vi "Gas_Setup.vi"() -> ()   [LabVIEW 2015]
uses:
  ADAM Controls/Ch_description_ADAM.ctl
  ADAM Controls/Module_type_ADAM.ctl
  ADAM Controls/Function_ADAM.ctl
  ADAM Controls/Channel_State.ctl
  ADAM Controls/Calib_type_ADAM.ctl
  ADAM Controls/Address.ctl
  ADAM Controls/Shut_Off_Valve.ctl
  ADAM Controls/Channel_names.ctl
  Channel_State_Control.ctl
  ADAM Controls/Update_scan_value.ctl
  Anemometry/Anemometry Sub Vis/Globals/Preference_global.vi
panel:
  out "Ch names":string[](array[string])
  in  "Select Plug Ins":bool
  in  "Source Info":string[][](table)
  in  "Carrier 1 Very Low":T1
  in  "Carrier 1 Hi-Tec Range":u16(ring) items=["Very Low", "Low", "High"]
  in  "Trace Hi-Tec Range":u16(ring) items=["5 ml/min", "50 ml/min", "300 ml/min"]
  in  "Carrier 1 High":T1
  in  "Carrier 1 Low":T1
  in  "300 ml/min":T1
  in  "5 ml/min":T1
  in  "Release Orientation":u16(ring) items=["Vertical", "Horizontal 0 Deg", "Downwards", "External System Tests", "Horizontal", "Edit Strings"]
  in  "Source Type":u16(ring) items=["11mm downward facing", "1mm Annulus above tank wall with Internal 2mm Annulus floating roof at 50mm.", "2 x ID=11mm Holes", "23mm IDD=8mm", "2mm Annulus around a quarter of inside of tank wall", "2mm Annulus around inside of tank wall", "4 point source ID=8.5mm located 90 deg apart on 8cm Diameter", "4 x 3mm holes spaced 8mm apart at roof perimeter", "70x70mm", "8  x 3mm holes spaced 10mm apart at roof perimeter", "8mm Annulus around inside of tank wall", "B2 D=6.8mm", "B204 Height 244mm ID 5.5mm", "B230 Height 152.4mm ID 8.5mm", "B30 Area", "B311 ID=11mm", "B331 ID=5.4mm", "B38_8mm_ID_passive", "B38_OD=3.1mm_ID=2mm", "B548 OD=13.8mm ID=3.5mm", "Both_Scrubbers_ID=4mm", "Both_Scrubbers_ID=7mm", "Capped release D=10mm H=10mm Slot=2mm", "D=12mm", "D=13.6mm", "D=16mm (ID=12 mm)", "D=18mm", "D=20mm", "D=22.5mm", "D=3.4mm", "D=5mm (ground release)", "D=6mm (ID=4.2 mm)", "D=7.1mm", "D=9mm", "D=9mm  20mm long passive", "Dext = 8.5 mm", "Exit Port of Solenoid Valve", "H=25:W=100mm", "H=50", "ID=1.6 OD=1.9", "ID=1.9 OD=3.0mm", "ID=103mm", "ID=15 mm 90 deg bend copper tube", "ID=20mm", "ID=24mm", "ID=3.4mm  OD= 4mm", "ID=3.9mm OD=6.3mm", "ID=4.25mm", "ID=4mm", "ID=5.1mm OD=5.8mm (Ground release)", "ID=5.1mm OD=5.8mm (roof release)", "ID=5.1mm at Z= 10mm  (Ground release)", "ID=50mm", "ID=5mm OD=5.8mm", "ID=6mm", "ID=6mm OD=8mm", "ID=7.75mm OD=10mm", "ID=8.6mm", "ID=8mm OD=9mm", "ID=9.2mm", "ID=9.5mm OD=12.5mm", "ID=9mm OD=10mm  Short Passive", "Line Source 100mm  1.07m width", "Line Source 25mm  1.3m long  perp to flow", "Line Source 25x1300", "Line Source 50mm  1.07m Wide", "Line source parallel to flow", "None", "Permeability_rig", "Pond_No1&2_140mm", "Pond_No1&2_84mm", "Pond_No1_84mm", "Pond_No2_84mm", "ROSE 9mm at last grid", "SAV ID=3.5mm", "Sample tubes in source", "Single 5mm Stack", "Single 7.9 mm stack", "THORP  ID=5.1mm", "Twin 5mm Stacks", "Twin Passive Stacks ID=8mm OD=8.7mm", "UKAEA ID=1.7mm", "W=50mm", "Edit Strings"]
  in  "Current Release Temp":dbl format="%.2f"
  in  "Release Temperature":u16(ring) items=["Enter Value", "A_Tunnel:Trav:1", "A_Tunnel:Speed:Dem Velocity", "A_Tunnel:Speed:Calib Tweak", "A_Tunnel:Speed:Dem Voltage", "A_Tunnel:Motor:Temp", "A_Tunnel:Motor:Enable", "A_Tunnel:Turbine:Enable", "A_Tunnel:Turbine_1:Dem_Volts", "A_Tunnel:Turbine_1:Dem_RPM", "Aero_Tunnel:Server:Pulse", "Aero_Tunnel:Motor:Temp", "Aero_Tunnel:Balance:Lift", "Aero_Tunnel:Balance:Pitch", "Aero_Tunnel:Balance:Drag", "Aero_Tunnel:Balance:Side-Force", "Aero_Tunnel:Balance:Yaw", "Aero_Tunnel:Balance:Roll", "B_Tunnel:Motor:Temp", "Cluster Room:General:Temp", "Cluster Room:Temp:Warning", "Complete:Scan:Period", "D_Tunnel:Motor:Temp", "EnFlo Lab:Hygrometry:Rel Humidity", "EnFlo Lab:Hygrometry:Dew Point temp", "EnFlo Lab:Hygrometry:Air Temp", "EnFlo Lab:labstrat1:Z=0m Floor", "EnFlo Lab:labstrat1:Z=0.1m", "EnFlo Lab:labstrat1:Z=0.5m", "EnFlo Lab:labstrat1:Z=1.5m", "EnFlo Lab:labstrat1:Z=2.5m", "EnFlo Lab:labstrat1:Z=3.5m", "EnFlo Lab:labstrat1:Z=4.5m", "EnFlo Lab:labstrat1:Z=5.75m Roof", "EnFlo Lab:labstrat1:Delta T", "EnFlo Lab:Desired:Air Temp", "EnFlo Lab:Heat:Extraction", "EnFlo Lab:labstrat1:Av Temp", "EnFlo Lab:Comp Air:Pressure", "EnFlo Lab:Emergency_Stop:Happy", "EnFlo Lab:Leak_Detector:Happy", "EnFlo Lab:Comp Air:Warning", "EnFlo_Tunnel:Speed:Dem Velocity", "EnFlo_Lab:Ventilation:Enable", "EnFlo_Lab:Window_Fans:Enable", "EnFlo_Lab:Window:Enable", "EnFlo_Lab:Window:Open", "EnFlo_Lab:West Window:Open1", "EnFlo_Lab:West Window:Open2", "EnFlo_Tunnel:Speed:Calib Tweak", "EnFlo_Tunnel:Speed:Dem Current", "EnFlo_Tunnel:Usonic:Velocity", "EnFlo_Tunnel:Usonic Y-ve Duct:Velocity", "EnFlo_Tunnel:Shaft:rpm", "EnFlo_Tunnel:Reference:Velocity", "EnFlo_Tunnel:Ref Pitot Pdyn SDP610:(Pa)", "EnFlo_Tunnel:Ref Pitot Zero SDP610:(Pa)", "EnFlo_Tunnel:Ref Pitot Zero:Enable", "EnFlo_Tunnel:Ref Pitot:Z (mm)", "EnFlo_Tunnel:Ref Pitot:Velocity", "EnFlo_Tunnel:Hydrosonic:Integral", "EnFlo_Tunnel:Days Run at:2.5m/s", "EnFlo_Tunnel:Floor_Cooling:Enable", "EnFlo_Tunnel:Heat_Ex_Div_Valve:Dem Pos", "EnFlo_Tunnel:Exit Duct:Dem Temp", "EnFlo_Tunnel:Exit Duct Top:Temp", "EnFlo_Tunnel:Exit Duct:Temp", "EnFlo_Tunnel:Chilled Water:Motor1 Temp", "EnFlo_Tunnel:Chilled Water:Motor2 Temp", "EnFlo_Tunnel:Chilled Water:Pressure_OK", "EnFlo_Tunnel:Chilled Water:Supply", "EnFlo_Tunnel:Chilled Water:Return", "EnFlo_Tunnel:Chilled Water:Dem Temp", "EnFlo_Tunnel:Chiller_Pump:Enable", "EnFlo_Tunnel:Chiller_Pump:Running", "EnFlo_Tunnel:Chilled Water:Valve Dem Pos", "EnFlo_Tunnel:Chilled Water:Valve Dem Voltage", "EnFlo_Tunnel:Chilled Water:Pressure_return (Bar)", "EnFlo_Tunnel:Chilled Water:Motor_Dem_Voltage", "EnFlo_Tunnel:Chilled Water:Desired_Delta_P", "EnFlo_Tunnel:Chilled Water:Pressure_supply (Bar)", "EnFlo_Tunnel:Fan Gearbox:Y+ Temp", "EnFlo_Tunnel:Fan Gearbox:Y- Temp", "EnFlo_Tunnel:Heater:Enable", "EnFlo_Tunnel:Motor:Enable", "EnFlo_Tunnel:Warning_Cone:Enable", "EnFlo_Tunnel:Tap_Water:Enable", "EnFlo_Tunnel:Pressure:Static", "EnFlo_Tunnel:P1:Enable", "EnFlo_Tunnel:P2:Enable", "EnFlo_Tunnel:P3:Enable", "EnFlo_Tunnel:P4:Enable", "EnFlo_Tunnel:P5:Enable", "EnFlo_Tunnel:K_Factor:1st_Honeycomb", "EnFlo_Tunnel:K_Factor:1st_Screen", "EnFlo_Tunnel:K_Factor:2nd_Screen", "EnFlo_Tunnel:K_Factor:2nd_Honeycomb_Heaters_Screen", "EnFlo_Tunnel:Inlet_Fan:Front_Trunk", "EnFlo_Tunnel:Inlet_Fan:Y-ve", "EnFlo_Tunnel:Inlet_Fan:Y+ve", "EnFlo_Tunnel:Inlet_Fan:Above Y-ve", "EnFlo_Tunnel:Inlet_Fan:Above Y=550", "EnFlo_Tunnel:Inlet_Fan:Above Y=1650", "EnFlo_Tunnel:Inlet_Fan:Upwards", "EnFlo_Tunnel:Motor:Temp", "EnFlo_Tunnel:Trav Origin:X Offset", "EnFlo_Tunnel:Trav Pos:X", "EnFlo_Tunnel:Trav Pos:Y", "EnFlo_Tunnel:Trav Pos:Z", "EnFlo_Tunnel:Temp:Pre_Inlet_Y=1500_Z=450", "EnFlo_Tunnel:Temp:Pre_Inlet_Y=-1500_Z=450", "EnFlo_Tunnel:Temp:Pre_Inlet_Y=1000_Z=450", "EnFlo_Tunnel:Temp:Pre_Inlet_Y=-1000_Z=450", "EnFlo_Tunnel:Temp:Pre_Inlet_Y=500_Z=450", "EnFlo_Tunnel:Temp:Pre_Inlet_Y=-500_Z=450", "EnFlo_Tunnel:Temp:Pre_Inlet_Y=0_Z=50", "EnFlo_Tunnel:Temp:Pre_Inlet_Y=0_Z=450", "EnFlo_Tunnel:Temp:Pre_Inlet_Y=0_Z=950", "EnFlo_Tunnel:Temp:Pre_Inlet_Y=0_Z=1450", "EnFlo_Tunnel:Temp:Pre_Inlet_Average", "EnFlo_Tunnel:Temp:Inlet_Y=0_Z=1450", "EnFlo_Tunnel:Temp:Inlet_Y=0_Z=1350", "EnFlo_Tunnel:Temp:Inlet_Y=0_Z=1250", "EnFlo_Tunnel:Temp:Inlet_Y=0_Z=1150", "EnFlo_Tunnel:Temp:Inlet_Y=0_Z=1050", "EnFlo_Tunnel:Temp:Inlet_Y=0_Z=950", "EnFlo_Tunnel:Temp:Inlet_Y=0_Z=850", "EnFlo_Tunnel:Temp:Inlet_Y=0_Z=750", "EnFlo_Tunnel:Temp:Inlet_Y=0_Z=650", "EnFlo_Tunnel:Temp:Inlet_Y=0_Z=550", "EnFlo_Tunnel:Temp:Inlet_Y=0_Z=450", "EnFlo_Tunnel:Temp:Inlet_Y=0_Z=350", "EnFlo_Tunnel:Temp:Inlet_Y=0_Z=250", "EnFlo_Tunnel:Temp:Inlet_Y=0_Z=150", "EnFlo_Tunnel:Temp:Inlet_Y=0_Z=50", "EnFlo_Tunnel:Temp:Inlet_Y=-1500_Z=1450", "EnFlo_Tunnel:Temp:Inlet_Y=-1500_Z=1350", "EnFlo_Tunnel:Temp:Inlet_Y=-1500_Z=1250", "EnFlo_Tunnel:Temp:Inlet_Y=-1500_Z=1150", "EnFlo_Tunnel:Temp:Inlet_Y=-1500_Z=1050", "EnFlo_Tunnel:Temp:Inlet_Y=-1500_Z=950", "EnFlo_Tunnel:Temp:Inlet_Y=-1500_Z=850", "EnFlo_Tunnel:Temp:Inlet_Y=-1500_Z=750", "EnFlo_Tunnel:Temp:Inlet_Y=-1500_Z=650", "EnFlo_Tunnel:Temp:Inlet_Y=-1500_Z=550", "EnFlo_Tunnel:Temp:Inlet_Y=-1500_Z=450", "EnFlo_Tunnel:Temp:Inlet_Y=-1500_Z=350", "EnFlo_Tunnel:Temp:Inlet_Y=-1500_Z=250", "EnFlo_Tunnel:Temp:Inlet_Y=-1500_Z=150", "EnFlo_Tunnel:Temp:Inlet_Y=-1500_Z=50", "EnFlo_Tunnel:Temp:Inlet_Y=-1000_Z=50", "EnFlo_Tunnel:Temp:Inlet_Y=-500_Z=50", "EnFlo_Tunnel:Temp:Inlet_Y=500_Z=50", "EnFlo_Tunnel:Temp:Inlet_Y=1000_Z=50", "EnFlo_Tunnel:Temp:Inlet_Y=1500_Z=50", "EnFlo_Tunnel:Temp:Inlet_Y=-1000_Z=450", "EnFlo_Tunnel:Temp:Inlet_Y=-500_Z=450", "EnFlo_Tunnel:Temp:Inlet_Y=500_Z=450", "EnFlo_Tunnel:Temp:Inlet_Y=1000_Z=450", "EnFlo_Tunnel:Temp:Inlet_Y=1500_Z=450", "EnFlo_Tunnel:Temp:Inlet_Y=-1000_Z=950", "EnFlo_Tunnel:Temp:Inlet_Y=-500_Z=950", "EnFlo_Tunnel:Temp:Inlet_Y=500_Z=950", "EnFlo_Tunnel:Temp:Inlet_Y=1000_Z=950", "EnFlo_Tunnel:Temp:Inlet_Y=1500_Z=950", "EnFlo_Tunnel:Temp:Inlet_Y=-1000_Z=1450", "EnFlo_Tunnel:Temp:Inlet_Y=-500_Z=1450", "EnFlo_Tunnel:Temp:Inlet_Y=500_Z=1450", "EnFlo_Tunnel:Temp:Inlet_Y=1000_Z=1450", "EnFlo_Tunnel:Temp:Inlet_Y=1500_Z=1450", "EnFlo_Tunnel:Inlet_Temp:Average", "EnFlo_Tunnel:Inlet_Temp:St Deviation", "EnFlo_Tunnel:Temp:Floor_Near_1", "EnFlo_Tunnel:Temp:Floor_Near_2", "EnFlo_Tunnel:Temp:Floor_Far_2", "EnFlo_Tunnel:Temp:Floor_Near_3", "EnFlo_Tunnel:Temp:Floor_Far_3", "EnFlo_Tunnel:Temp:Floor_Near_4", "EnFlo_Tunnel:Temp:Floor_Far_4", "EnFlo_Tunnel:Temp:Floor_Near_5", "EnFlo_Tunnel:Temp:Floor_Far_5", "EnFlo_Tunnel:Temp:Floor_Near_6", "EnFlo_Tunnel:Temp:Floor_Far_6", "EnFlo_Tunnel:Temp:Floor_Near_7", "EnFlo_Tunnel:Temp:Floor_Far_7", "EnFlo_Tunnel:Temp:Floor_Near_8", "EnFlo_Tunnel:Temp:Floor_Far_8", "EnFlo_Tunnel:Temp:Floor_Near_12", "EnFlo_Tunnel:Temp:Floor_Far_12", "EnFlo_Tunnel:Temp:Z=50_Y=1415", "EnFlo_Tunnel:Therm:Master_Reference", "EnFlo_Tunnel:Temp:Floor_11.3", "EnFlo_Tunnel:Temp:Floor_12.1", "EnFlo_Tunnel:Temp:Y+ve_Side_Top", "EnFlo_Tunnel:Temp:Y+ve_Side_Middle", "EnFlo_Tunnel:Temp:Y+ve_Side_Bottom", "EnFlo_Tunnel:Temp:Y-ve_Side_Top", "EnFlo_Tunnel:Temp:Y-ve_Side_Middle", "EnFlo_Tunnel:Temp:Y-ve_Side_Bottom", "EnFlo_Tunnel:Temp:Y+ve_Side_Flow_Top", "EnFlo_Tunnel:Temp:Y+ve_Side_Flow_Middle", "EnFlo_Tunnel:Temp:Y+ve_Side_Flow_Bottom", "EnFlo_Tunnel:Temp:Y-ve_Side_Flow_Top", "EnFlo_Tunnel:Temp:Y-ve_Side_Flow_Middle", "EnFlo_Tunnel:Temp:Y-ve_Side_Flow_Bottom", "EnFlo_Tunnel:Temp:Roof_Far_2", "EnFlo_Tunnel:Temp:Roof_Near_3", "EnFlo_Tunnel:Temp:Roof_Far_4", "EnFlo_Tunnel:Temp:Roof_Far_6", "EnFlo_Tunnel:Temp:Roof_Near_7", "EnFlo_Tunnel:Temp:Roof_Far_8", "EnFlo_Tunnel:Temp:Roof_Far_10", "EnFlo_Tunnel:Temp:Roof_Near_12", "EnFlo_Tunnel:Temp:Roof_Far_15", "EnFlo_Tunnel:Temp:Roof_Far_19", "EnFlo_Tunnel:Temp:LDA Probe", "EnFlo_Tunnel:Cold_Wire:Therm", "EnFlo_Tunnel:FFID:Temp", "EnFlo_Tunnel:FFID2:Temp", "Spirit_Smoke:Generator:Enable", "Spirit_Smoke:Generator Puff:Enable", "EnFlo_Tunnel:Lights:Enable", "EnFlo_Tunnel:Trav1 Pos:Z", "EnFlo_Tunnel:Trav1 Pos:Y", "EnFlo_Tunnel:Trav1 Pos:X", "EnFlo_Tunnel:Trav2 Pos:Z", "EnFlo_Tunnel:Trav2 Pos:Y", "EnFlo_Tunnel:Trav2 Pos:X", "EnFlo_Tunnel:Source_Pos:Z", "EnFlo_Tunnel:Safety_Loop:Status", "EnFlo_Tunnel:Gas Solenoid:Status", "EnFlo_Tunnel:Source1:Enable", "EnFlo_Tunnel:Source2:Enable", "EnFlo_Tunnel:Source3:Enable", "EnFlo_Tunnel:Source_Pos:X_Model", "EnFlo_Tunnel:Source_Pos:Y_Model", "EnFlo_Tunnel:Job:Name", "EnFlo_Tunnel:Obstacle/:Building", "EnFlo_Tunnel:Vorticity:Generators", "EnFlo_Tunnel:Roughness:Height", "EnFlo_Tunnel:Side Wall:Separation", "EnFlo_Tunnel:Safety:GMU_Watchdog", "FFID:System:Enable", "Froude:NPL:Atmos_Press", "GMU:Source:Type", "GMU:Release:Orientation", "GMU:Trace:Gas", "GMU:Carrier 1:Gas", "GMU:Carrier 2:Gas", "GMU:Carrier 1:Hi-Tec Range", "GMU:Trace:Hi-Tec Range", "GMU:Carrier 1:Dem Volt", "GMU:Carrier 2:Dem Volt", "GMU:Trace:Dem Volt", "Clean_Air:Hi-Tec:Dem Volt", "GMU:Carrier 1:Meas Volt", "GMU:Carrier 2:Meas Volt", "GMU:Trace:Meas Volt", "Clean_Air:Hi-Tec:Meas Volt", "GMU:Carrier 1:Meas Q", "GMU:Carrier 2:Meas Q", "GMU:Trace:Meas Q", "GMU:Carrier 1:Meas M_dot", "GMU:Carrier 2:Meas M_dot", "GMU:Trace:Meas M_dot", "GMU:Remaining:Nitrogen", "GMU:Remaining:Helium", "GMU:Remaining:CO2", "GMU:Remaining:Krypton", "GMU:Remaining:Ethane", "GMU:Remaining:Propane", "GMU:Calibration:Gas 1", "GMU:Calibration:Gas 2", "GMU:Carrier 1:Dem Q", "GMU:Carrier 2:Dem Q", "GMU:Trace:Dem Q", "GMU:Source:Dem Q", "GMU:Source:Meas Q", "GMU:Source:Meas M_dot", "GMU:Source:Meas Density", "GMU:Source:Meas Den Ratio", "GMU:Source:Dem Strength", "GMU:Source:ppm/%Density", "GMU:Source:Meas Strength", "GMU:Source:Est Time", "GMU:Detector:Meas Current", "GMU:Detector:Strength", "GMU:Test:Ethane trip", "GMU:Source:Release Temp", "GMU:Gas:Enable", "GMU:Detector:Happy", "GMU:Source:Pressure", "GMU:Trace:Open", "GMU:CO2_Rig:Enable", "GMU:CO2_Supply:Pressure (Bar)", "GMU:CO2_Bath:Temp", "GMU:Mixing_Pipe:Temp", "Hydrosonic:Transducer:Setting", "Hydrosonic:Seeder:Enable", "Laser:Power Meter:Reading (mW)", "LDA1:System:Enable", "LDA2:Tank:Supply Temp", "LDA2:System:Enable", "Uni:Chilled Water:Temp", "University:Outside:Temp", "University:Chilled Water:Requested", "A_Tunnel:Probe:Roll", "A_Tunnel:Pitot:Velocity", "A_Tunnel::Velocity", "A_Tunnel:Probe:Yaw", "A_Tunnel:Probe:Pitch", "EnFlo Lab:ScaniValve:Combined_Position", "A_Tunnel:Wing:Pitch", "EnFlo_Tunnel:Seeder_Pump:Enable", "EnFlo_Tunnel:Seeder:High_Flow", "EnFlo_Tunnel:Seeder:Low_Flow", "EnFlo_Tunnel:Seeder_Fridge:Temp", "EnFlo_Tunnel:Seeder:Power", "GMU:Source:Gas", "Tank:Depth:mm", "Tank:Fill_Valve:Enable", "Tank:Fill:Now", "Tank:Desired_Depth:mm", "Tank:Water:Temp", "GMU:CO2_Low:Siren", "A_Tunnel:Trav Pos:Z", "A_Tunnel:Trav Pos:Y", "A_Tunnel:Trav Pos:X", "EnFlo_Stack:Floor:Surface (mm)", "EnFlo Lab:Hygrometry:Rel Humidity_PN", "EnFlo Lab:Hygrometry:Atmos_Press_PN", "EnFlo Lab:Hygrometry:Air Temp_PN", "EnFlo Lab:Hygrometry:Dew Point temp_PN", "EnFlo_Tunnel Metadata:Probe_Setup:Time", "GMU:Source:Live", "GMU:Back_Press_Valve:Volts", "GMU:Back_Press_Valve:Position", "EnFlo_Tunnel:Usonic_Ref_3:Velocity", "EnFlo_Tunnel:Usonic_Ref_3:Direction", "EnFlo_Tunnel:Temp:Pre_Inletx_Ch1", "EnFlo_Tunnel:Trav3 Pos:X", "EnFlo_Tunnel:Trav3 Pos:Z", "EnFlo_Tunnel:Trav3 Pos:Y", "EnFlo_Lab:Window_Fans:Power_%", "EnFlo_Tunnel:Trav_Blockage_Fans:Desired_Volts", "EnFlo_Tunnel:Trav_Blockage_Fans:Meas_Volts", "EnFlo_Tunnel:Trav_Blockage_Fans:Demand_%", "EnFlo_Tunnel:Heater:Dem Volts", "EnFlo_Tunnel:Heater:Dem Power", "EnFlo_Tunnel:Wind:Direction Deg", "EnFlo_Tunnel:Chiller_Pump_Floor:Dem_Power(%)", "EnFlo_Tunnel:Chiller_Pump_Exchanger:Dem_Power(%)", "EnFlo_Tunnel:Exit_Heaters:Dem_Power(%)", "EnFlo_Tunnel Metadata:Screens_Downstream:of Heaters", "EnFlo_Tunnel Metadata:Roughness Elements:1st Row X(m)", "EnFlo_Tunnel:Wind_Turbine:Enable", "EnFlo_Tunnel:De-humidifier:Current_Clamp", "A_Tunnel:Heater_Mat:Enable", "EnFlo_Tunnel:Trav4 Pos:Z", "EnFlo_Tunnel Metadata:2nd_Honeycombe:Upstream of heaters", "GMU:Mains Divertor:Valve", "Status:of:Post_Processing_Machine", "Status:of:ADAM_Server", "Status:of:EnFlo_Tunnel", "Status:of:Aero_Tunnel", "Status:of:A_Tunnel", "EnFlo_Tunnel:Source:Status", "GMU:Trace_2:Dem Volt", "GMU:Trace_2:Meas Volt", "Status:of:Paul_Hayden_Desk"]
  in  "Gas Remaining":string[][](table)
  in  "Calib 2":dbl format="%.2f"
  in  "Calib 1":dbl format="%.2f"
  in  "Carrier 2 Gas":u16(ring) items=["Air", "Nitrogen", "Helium", "CO2", "Krypton", "None"]
  in  "Trace Gas":u16(ring) items=["Propane", "Ethane"]
  in  "Carrier 1 Gas":u16(ring) items=["Air", "Nitrogen", "Helium", "CO2", "Krypton", "None"]
  out "Numerical Values":dbl[](array[numeric]) format="%.9f"
  out "Ch Description Array":T2[](array[typedef]) {"Duty" format="%.0b"; "D" format="%#_5g"; "C" format="%#_5g"; "B" format="%#_5g"; "A" format="%#_5g"}
  out "dup reference":refnum<vi>
  in  "stop":bool
  in  "OK":bool
  # "Calibration Gas (ppm)"
  # "300\nml/min"
  # "5\nml/min"
  # "50\nml/min"
  # "Low\nRange"
  # "Very\nLow\nRange"
  # "High\nRange"
  # "Dispersion Setup"
  # "To Source"
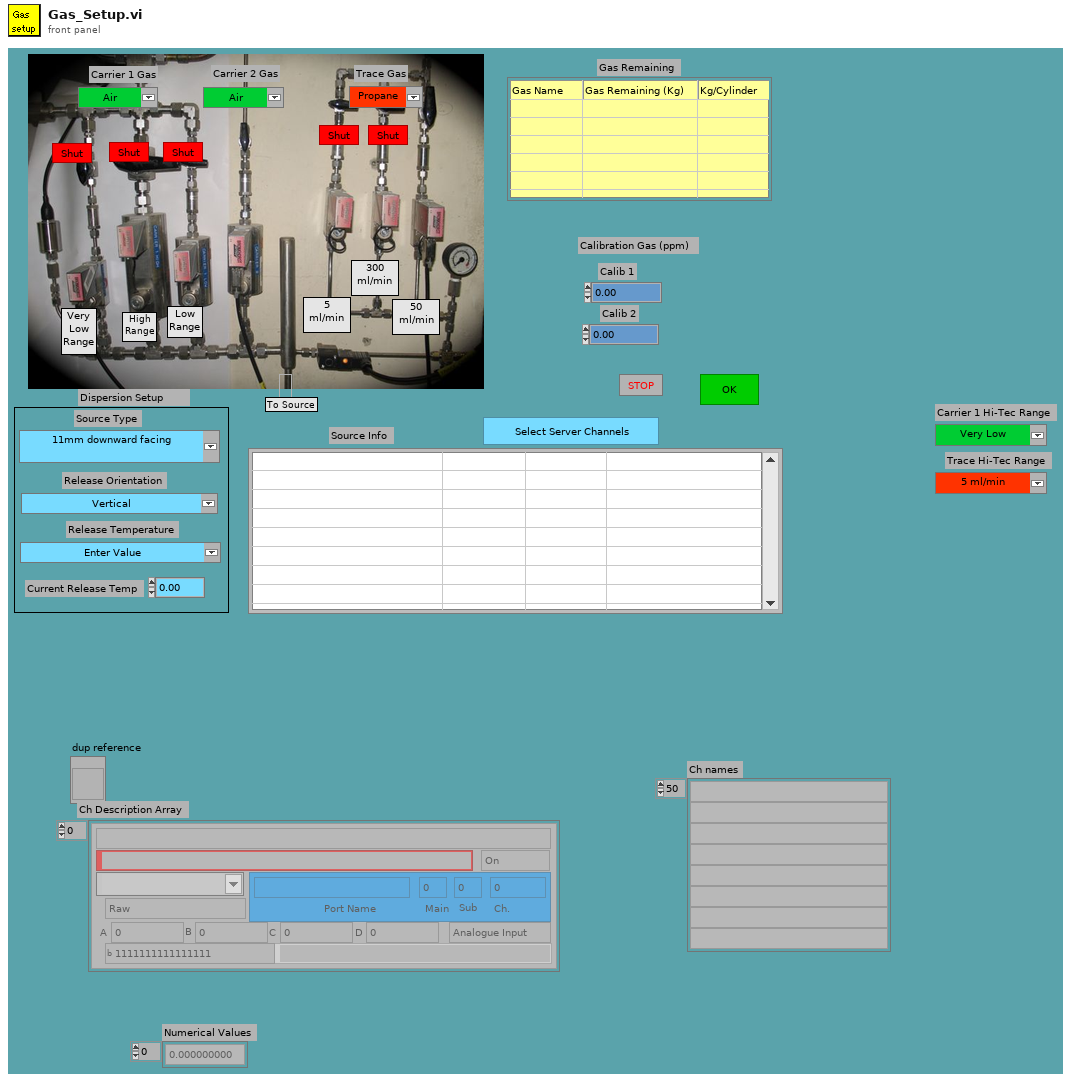
[diagram p1: front panel]
types:
  T1 = typedef "Shut_Off_Valve.ctl" = bool
  T2 = typedef "Ch_description_ADAM.ctl" = cluster{"Ch Name":string, "Type":T3, "Function":T4, "Ch State":T5, "Calibration type":T6, "A":dbl, "B":dbl, "C":dbl, "D":dbl, "Comments":string, "Address":T7, "String":string, "Duty":u16}
  T3 = typedef "Module_type_ADAM.ctl" = string
  T4 = typedef "Function_ADAM.ctl" = enum16{"Analogue Input", "Digital Input", "Event counter", "Event rate", "Analogue Output", "Digital Output", "Relay Output"}
  T5 = typedef "Channel_State.ctl" = enum16{"On", "Off", "Always On", "Always Off"}
  T6 = typedef "Calib_type_ADAM.ctl" = enum16{"Raw", "Bx + A", "Cx^2 + Bx + A", "Dx^3 + Cx^2 + Bx + A", "In Band", "Hi-Tec Q", "Hi-Tec M_dot", "Text"}
  T7 = typedef "Address.ctl" = cluster{"Main":i32, "Ch.":i32, "Sub":i32, "Port Name":string}
  T8 = typedef "Channel_names.ctl" = enum16{"Active Only", "Active + Off", "All Channels"}
  T9 = typedef "Channel_State_Control.ctl" = enum16{"Channel Name", "Channel Name Starts with", "Main Address"}
  T10 = typedef "Update_scan_value.ctl" = cluster{"Channel Name":string, "New Value":dbl}
  T11 = enum16{"Zero or one", "One", "Zero or more", "One or more"}
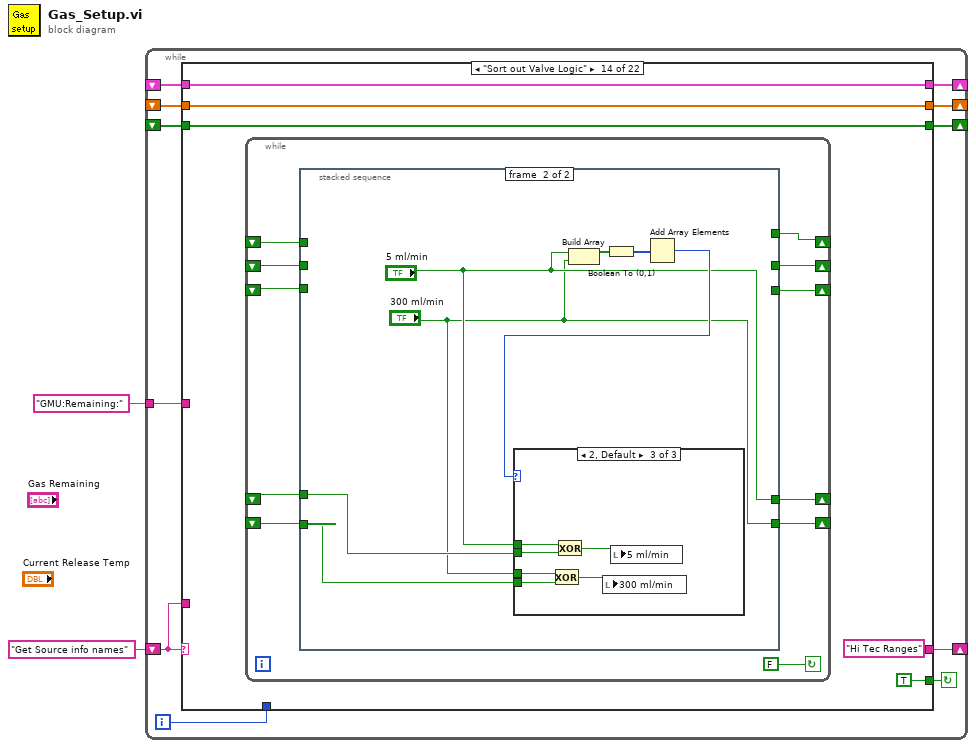
[diagram p0: block diagram]
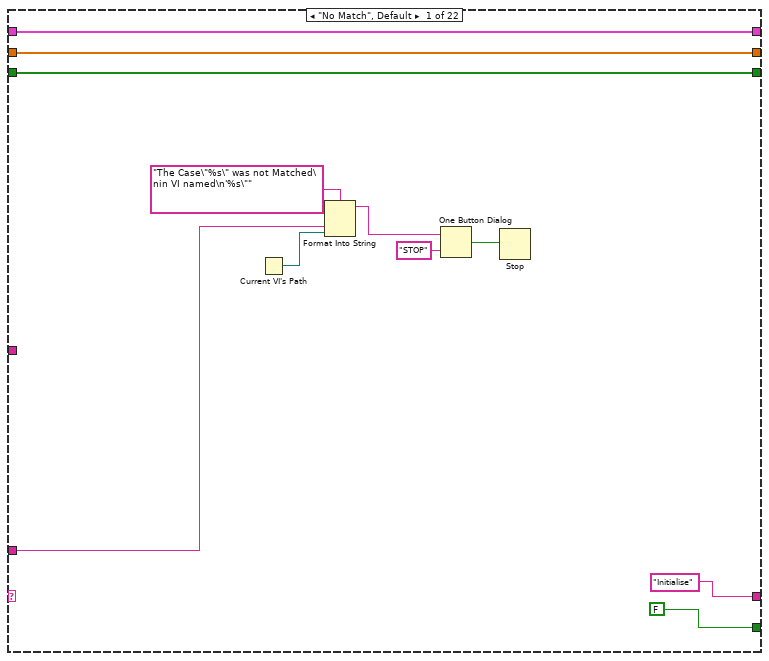
[diagram p2: hidden frame]
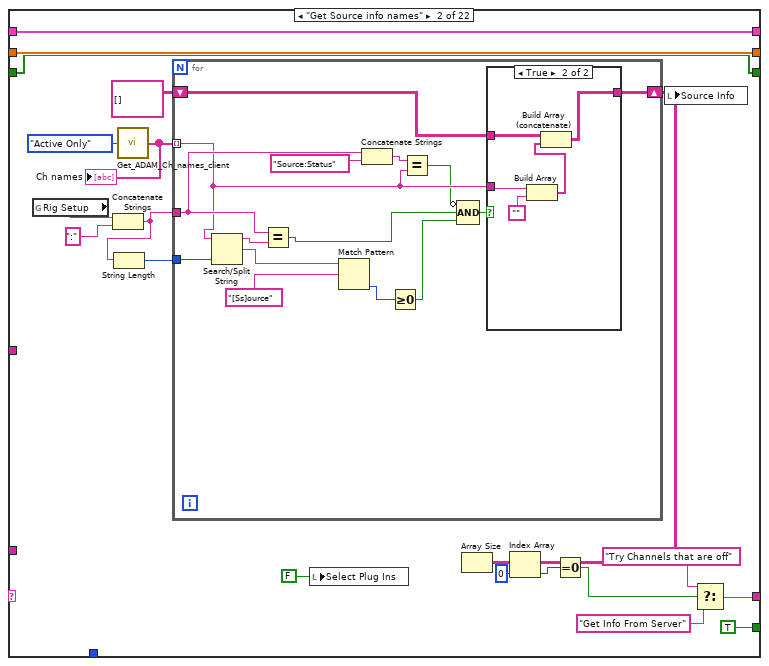
[diagram p3: hidden frame]
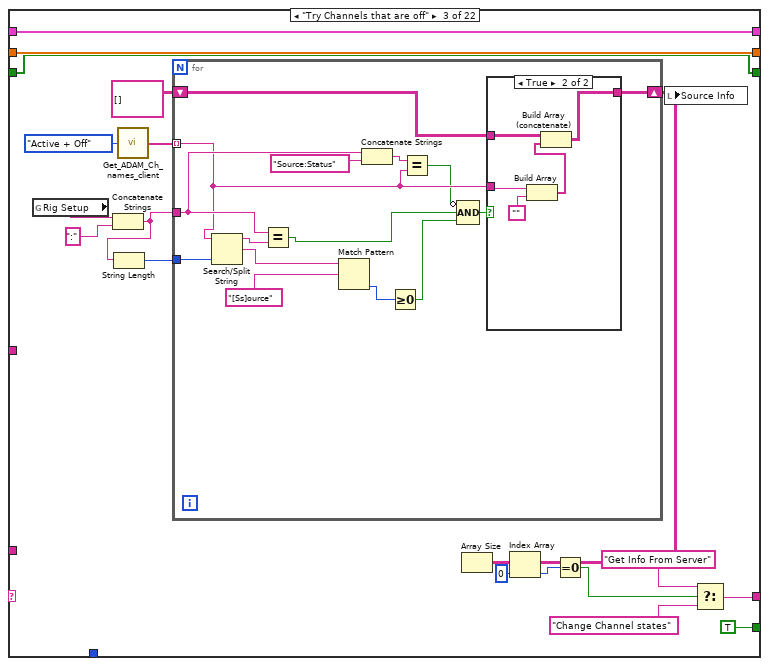
[diagram p5: hidden frame]
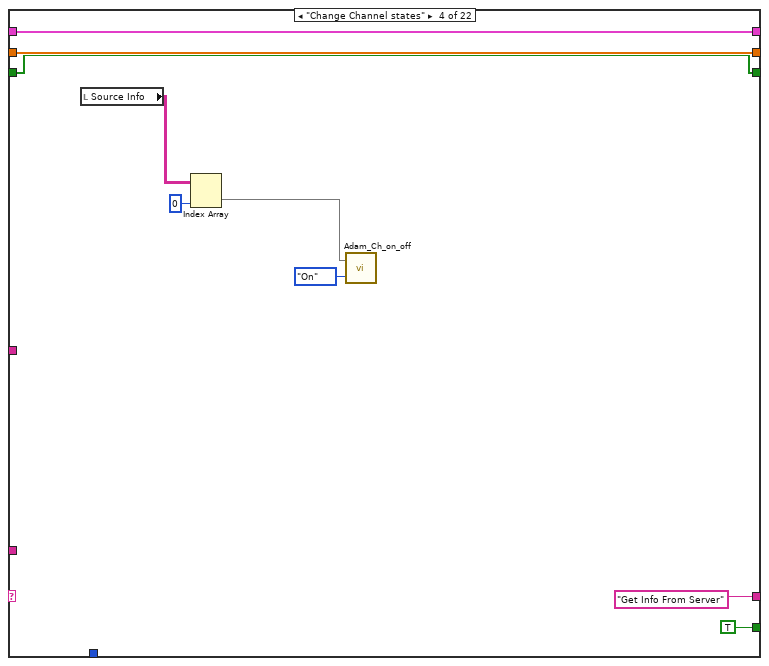
[diagram p7: hidden frame]
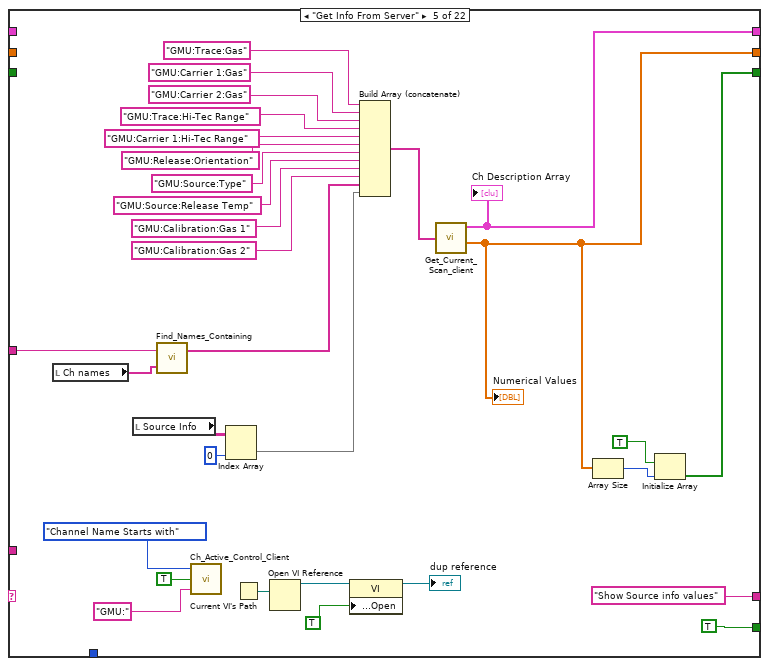
[diagram p8: hidden frame]
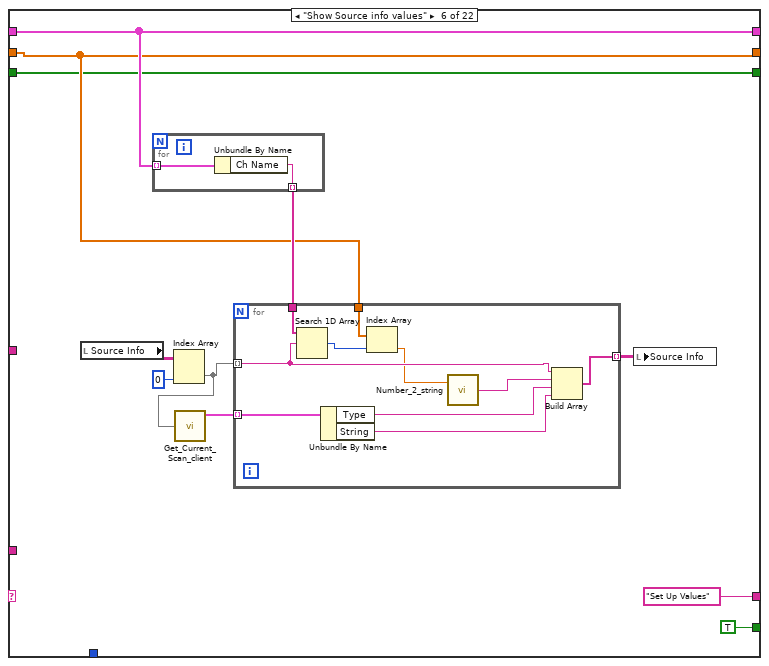
[diagram p9: hidden frame]
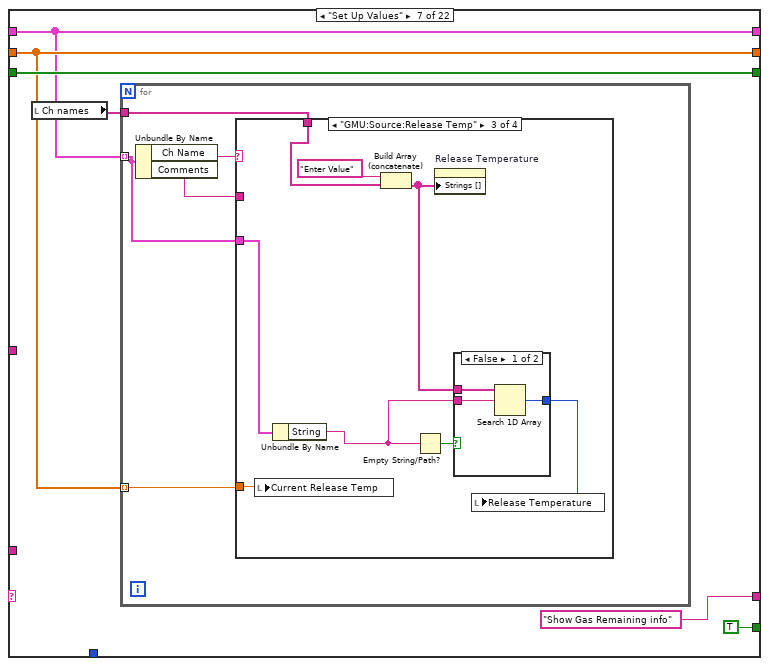
[diagram p10: hidden frame]
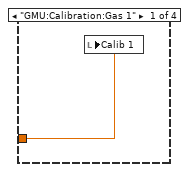
[diagram p11: hidden frame]
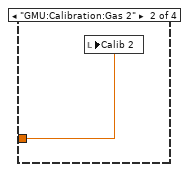
[diagram p12: hidden frame]
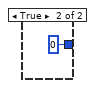
[diagram p13: hidden frame]
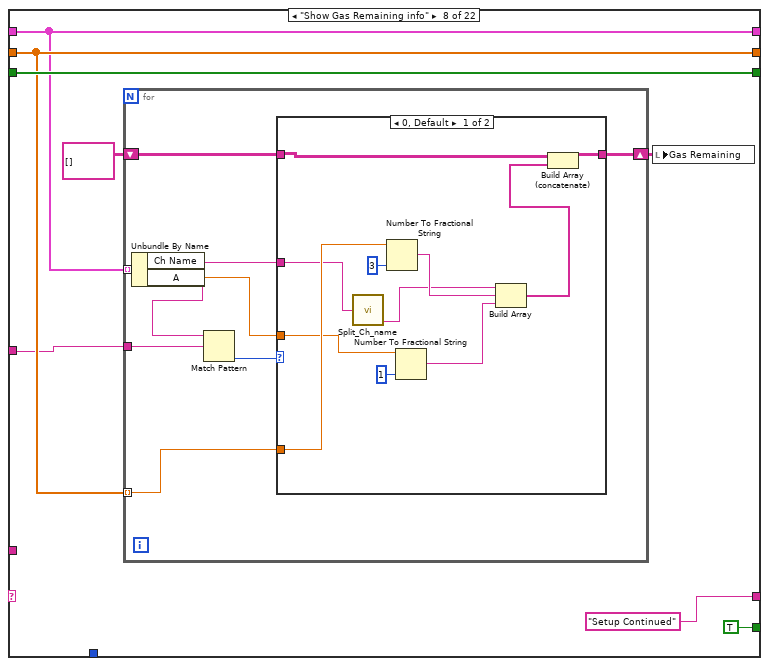
[diagram p15: hidden frame]
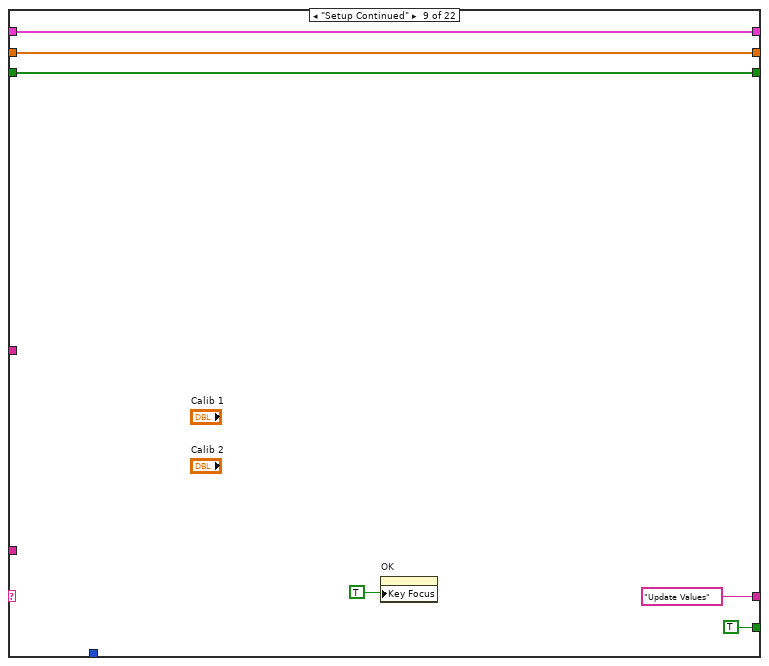
[diagram p17: hidden frame]
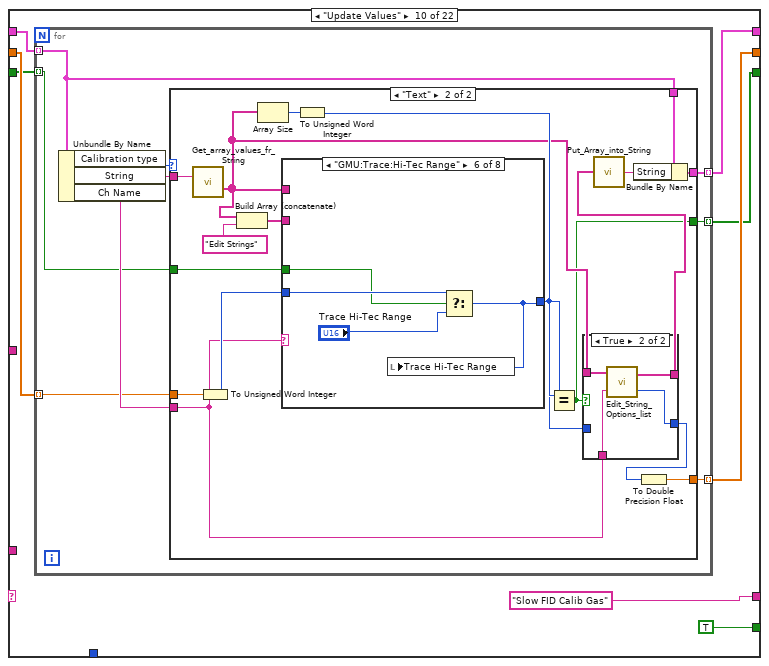
[diagram p18: hidden frame]
diagram:
  n1 = while {
    shift-left: _ -> [w5]
    shift-right: [w6] -> _
    shift-left: _ -> [w7]
    shift-right: [w9] -> _
    shift-left: _ -> [w8]
    shift-right: [w10] -> _
    shift-left: "Get Source info names" ("t") -> [w11]
    shift-right: [w12] -> _
    tunnel: "GMU:Remaining:" -> [w3]
    i -> [w4]
    stop <- w13 continue-if-true
    n2 = case shown="\"Sort out Valve Logic\"" w11 {
      tunnel: [FALSE TRUE ("T button?") TRUE ("T button?") TRUE ("T button?") TRUE TRUE ("T button?") TRUE ("T button?") TRUE ("T button?") TRUE ("T button?") TRUE ("T button?") TRUE ("T button?") TRUE ("T button?") TRUE ("T button?") TRUE ("T button?") TRUE ("T button?") TRUE ("T button?") TRUE ("T button?") TRUE ("T button?") TRUE ("T button?") TRUE ("T button?") TRUE ("T button?") FALSE ("T button?")] -> w13
      tunnel: ["Initialise" w26 w68 "Get Info From Server" "Show Source info values" "Set Up Values" "Show Gas Remaining info" "Setup Continued" "Update Values" "Slow FID Calib Gas" w311 "Update Release Temperature" "Sort out Valve Logic" "Hi Tec Ranges" "Continue looping?" w435 "Insert Gas Remaining Info" "Insert Source info values" "Update Server" w531 "Get Source info names" ("t") "End"] -> w12
      tunnel: w11 -> [w19 _ _ _ _ _ _ _ _ _ _ _ _ _ _ _ _ _ _ _ _ _]
      tunnel: [w16 w40 w80 w114 w138 w155 w170 w197 w227 w233 w315 w327 w354 w371 w422 w441 w443 w480 w512 w540 w596 w647] -> w10
      tunnel: [w15 w39 w79 w113 w125 w154 w171 w198 w226 w231 w314 w326 w353 w370 w421 w440 w446 w486 w514 w539 w595 w646] -> w9
      tunnel: w8 -> [w16 w40 w80 w114 _ w155 w170 w197 w227 w234 w315 w327 w354 w371 w422 w441 w444 w480 w512 w540 w596 w647]
      tunnel: w7 -> [w15 w39 w79 w113 _ w154 w171 w198 w226 w232 w314 w326 w353 w370 w421 w440 w445 w485 w515 w539 w595 w646]
      tunnel: [w14 w38 w78 w112 w124 w153 w173 w200 w224 w228 w309 w324 w351 w368 w419 w434 w448 w488 w511 w538 w594 w639] -> w6
      tunnel: w5 -> [w14 w38 w78 w112 _ w153 w173 w200 w224 w229 w309 w324 w351 w368 w419 w434 w448 w488 w511 w538 w594 w639]
      tunnel: w4 -> [_ _ _ _ _ _ _ _ _ _ w308 _ _ _ _ _ _ _ _ _ _ _]
      tunnel: w3 -> [_ _ _ _ w122 _ _ w196 _ _ _ _ _ _ _ _ _ w479 _ _ _ _]
      frame "No Match", Default {
        n3 = Current VI's Path() -> (path=w18:path)
        n4 = Format Into String(format string="The Case\"%s\" was not Matched\nin VI named\n'%s\"" ("Format String"), w19, w18) -> (resulting string=w22:string)  [unwired: 2 in, 1 out]
        n5 = One Button Dialog(message=w22, button name ("OK")="STOP") -> (true=w20:bool)
        n6 = Stop(stop? (T)=w20) -> ()
      }
      frame "Get Source info names" {
        n7 = global read "Preference_global.vi" "Rig Setup"() -> (w44:string)
        n8 = Concatenate Strings(w44, ":" ("string")) -> (w41:string)
        n9 = String Length(string=w41) -> (length=w42:i32)
        n10 = call "Get_ADAM_Ch_names_client.vi"("Channel names set"=Channel_names."Active Only") -> ("Ch names"=w35:string[])
        "Ch names" <- w35
        n11 = for {
          tunnel: w42 -> [w59]
          tunnel: w35 -> [w49] mode=indexing
          tunnel: w41 -> [w51]
          shift-right: [w53] -> w33
          shift-left: string[][] [] -> [w54]
          n12 = Search/Split String(string=w49, offset (0)=w59) -> (substring before match=w58:string, match + rest of string=w57:string)  [unwired: 2 out]
          n13 = Equal?(x=w51, y=w58) -> (x = y?=w47:bool)
          n14 = Match Pattern(string=w57, regular expression="[Ss]ource") -> (offset past match=w55:i32)  [unwired: 4 out]
          n15 = Concatenate Strings(w51, "Source:Status") -> (w50:string)
          n16 = Greater Or Equal To 0?(x=w55) -> (x >= 0?=w48:bool)
          n17 = Equal?(x=w50, y=w49) -> (x = y?=w46:bool)
          n18 = Compound Arithmetic op=AND(invert w46, w47, w48) -> (w45:bool)
          n19 = case shown="True" w45 {
            tunnel: w54 -> [w60 w65]
            tunnel: w49 -> [_ w63]
            tunnel: [w60 w64] -> w53
            frame False {
            }
            frame True {
              n20 = Build Array(w63, "") -> (w61:string[])
              n21 = Build Array (concatenate)(w65, w61) -> (w64:string[][])
            }
          }
        }
        n22 = local write "Select Plug Ins"(FALSE ("Select Plug Ins")) -> ()
        n23 = Array Size(array=w33) -> (size(s)=w32:i32[])
        n24 = Index Array(array=w32, index=0) -> (element=w30:i32)
        n25 = Equal To 0?(x=w30) -> (x = 0?=w28:bool)
        n26 = local write "Source Info"(w33) -> ()
        n27 = Select(t="Try Channels that are off", s=w28, f="Get Info From Server") -> (s? t:f=w26:string)
      }
      frame "Try Channels that are off" {
        n28 = global read "Preference_global.vi" "Rig Setup"() -> (w84:string)
        n29 = Concatenate Strings(w84, ":" ("string")) -> (w81:string)
        n30 = String Length(string=w81) -> (length=w82:i32)
        n31 = call "Get_ADAM_Ch_names_client.vi"("Channel names set"=Channel_names."Active + Off") -> ("Ch names"=w75:string[])
        n32 = for {
          tunnel: w82 -> [w99]
          tunnel: w75 -> [w89] mode=indexing
          tunnel: w81 -> [w91]
          shift-right: [w93] -> w74
          shift-left: string[][] [] -> [w94]
          n33 = Search/Split String(string=w89, offset (0)=w99) -> (substring before match=w98:string, match + rest of string=w97:string)  [unwired: 2 out]
          n34 = Equal?(x=w91, y=w98) -> (x = y?=w87:bool)
          n35 = Match Pattern(string=w97, regular expression="[Ss]ource") -> (offset past match=w95:i32)  [unwired: 4 out]
          n36 = Concatenate Strings(w91, "Source:Status") -> (w90:string)
          n37 = Greater Or Equal To 0?(x=w95) -> (x >= 0?=w88:bool)
          n38 = Equal?(x=w90, y=w89) -> (x = y?=w86:bool)
          n39 = Compound Arithmetic op=AND(invert w86, w87, w88) -> (w85:bool)
          n40 = case shown="True" w85 {
            tunnel: w94 -> [w100 w105]
            tunnel: w89 -> [_ w103]
            tunnel: [w100 w104] -> w93
            frame False {
            }
            frame True {
              n41 = Build Array(w103, "") -> (w101:string[])
              n42 = Build Array (concatenate)(w105, w101) -> (w104:string[][])
            }
          }
        }
        n43 = Array Size(array=w74) -> (size(s)=w73:i32[])
        n44 = Index Array(array=w73, index=0) -> (element=w71:i32)
        n45 = Equal To 0?(x=w71) -> (x = 0?=w69:bool)
        n46 = local write "Source Info"(w74) -> ()
        n47 = Select(t="Get Info From Server", s=w69, f="Change Channel states") -> (s? t:f=w68:string)
      }
      frame "Change Channel states" {
        n48 = local read "Source Info"() -> (w109:string[][])
        n49 = Index Array(array=w109, index (col)=0 ("disabled index (col)")) -> (element=w107:string[])  [unwired: 1 in]
        n50 = call "Adam_Ch_on_off.vi"("Ch State"=Channel_State."On", "ADAM Ch Names"=w107) -> ()  [unwired: 1 out]
      }
      frame "Get Info From Server" {
        n51 = local read "Ch names"() -> (w115:string[])
        n52 = local read "Source Info"() -> (w118:string[][])
        n53 = call "Find_Names_Containing.vi"("Ch names"=w115, "String to match"=w122) -> ("Matched Names"=w123:string[])  [unwired: 1 out]
        n54 = call "Ch_Active_Control_Client.vi"("Match"="GMU:", "Activate Channels?"=TRUE, "Control on"=Channel_State_Control."Channel Name Starts with") -> ()  [unwired: 2 out]
        n55 = Index Array(array=w118, index (col)=0 ("disabled index (col)")) -> (element=w116:string[])  [unwired: 1 in]
        n56 = Current VI's Path() -> (path=w140:path)
        n57 = Open VI Reference(vi path=w140) -> (vi reference=w141:refnum<vi>)  [unwired: 1 in, 5 out]
        n58 = property class="VI"(reference=w141, "Front Panel Window:Open"=TRUE) -> (reference out=→"dup reference":refnum<vi>)  [unwired: 1 in, 1 out]
        n59 = Build Array (concatenate)("GMU:Trace:Gas", "GMU:Carrier 1:Gas", "GMU:Carrier 2:Gas", "GMU:Trace:Hi-Tec Range", "GMU:Carrier 1:Hi-Tec Range", "GMU:Release:Orientation", "GMU:Source:Type", "GMU:Source:Release Temp", "GMU:Calibration:Gas 1", "GMU:Calibration:Gas 2", w123, w116) -> (w143:string[])
        n60 = call "Get_Current_Scan_client.vi"("ADAM Ch Names"=w143) -> ("Ch Description Array"=w138:T2[], "Numerical Values"=w125:dbl[])  [unwired: 2 out]
        "Ch Description Array" <- w138
        "Numerical Values" <- w125
        n61 = Array Size(array=w125) -> (size(s)=w127:i32)
        n62 = Initialize Array(TRUE, w127) -> (w124:bool[])
      }
      frame "Show Source info values" {
        n63 = local read "Source Info"() -> (w149:string[][])
        n64 = for {
          tunnel: w155 -> [w168] mode=indexing
          tunnel: [w167] -> w156 mode=indexing
          n65 = Unbundle By Name(w168) -> ("Ch Name"=w167:string)
        }
        n66 = Index Array(array=w149, index (col)=0 ("disabled index (col)")) -> (element=w147:string[])  [unwired: 1 in]
        n67 = call "Get_Current_Scan_client.vi"("ADAM Ch Names"=w147) -> ("Ch Description Array"=w146:T2[])  [unwired: 1 in, 2 out]
        n68 = for {
          tunnel: w156 -> [w166]
          tunnel: w147 -> [w163] mode=indexing
          tunnel: w154 -> [w164]
          tunnel: [w160] -> w152 mode=indexing
          tunnel: w146 -> [w159] mode=indexing
          n69 = Search 1D Array(1D array=w166, element=w163) -> (index of element=w165:i32)  [unwired: 1 out]
          n70 = Unbundle By Name(w159) -> ("Type"=w158:T3, "String"=w157:string)
          n71 = Index Array(array=w164, index=w165) -> (element=w162:dbl)
          n72 = call "Number_2_string.vi"("number"=w162) -> ("String"=w161:string)  [unwired: 1 in]
          n73 = Build Array(w163, w161, w158, w157) -> (w160:T3[])
        }
        n74 = local write "Source Info"(w152) -> ()
      }
      frame "Set Up Values" {
        n75 = local read "Ch names"() -> (w169:string[])
        n76 = for {
          tunnel: w171 -> [w175] mode=indexing
          tunnel: w170 -> [w177] mode=indexing
          tunnel: w169 -> [w176]
          n77 = Unbundle By Name(w177) -> ("Ch Name"=w179:string, "Comments"=w178:string)
          n78 = case shown="\"GMU:Source:Release Temp\"" w179 {
            tunnel: w175 -> [w180 w181 w185 _]
            tunnel: w178 -> [_ _ _ _]
            tunnel: w177 -> [_ _ w189 _]
            tunnel: w176 -> [_ _ w183 _]
            frame "GMU:Calibration:Gas 1" {
              n79 = local write "Calib 1"(w180) -> ()
            }
            frame "GMU:Calibration:Gas 2" {
              n80 = local write "Calib 2"(w181) -> ()
            }
            frame "GMU:Source:Release Temp" {
              n81 = local write "Current Release Temp"(w185) -> ()
              n82 = Unbundle By Name(w189) -> ("String"=w187:string)
              n83 = Build Array (concatenate)("Enter Value", w183) -> (w182:string[])
              n84 = Empty String/Path?(string/path=w187) -> (empty?=w188:bool)
              n85 = property on="Release Temperature" class="Ring (strict)"("Strings []"=w182) -> ()  [unwired: 2 in, 2 out]
              n86 = case shown="False" w188 {
                tunnel: w182 -> [w192 _]
                tunnel: w187 -> [w191 _]
                tunnel: [w190 0 ("index of element")] -> w186
                frame False {
                  n87 = Search 1D Array(1D array=w192, element=w191) -> (index of element=w190:i32)  [unwired: 1 out]
                }
                frame True {
                }
              }
              n88 = local write "Release Temperature"(w186) -> ()
            }
            frame "No Match", Default {
            }
          }
        }
      }
      frame "Show Gas Remaining info" {
        n89 = for {
          tunnel: w198 -> [w204] mode=indexing
          tunnel: w197 -> [w209] mode=indexing
          tunnel: w196 -> [w208]
          shift-right: [w205] -> w194
          shift-left: string[][] [] -> [w206]
          n90 = Unbundle By Name(w209) -> ("Ch Name"=w202:string, "A"=w203:dbl)
          n91 = Match Pattern(string=w202, regular expression=w208) -> (offset past match=w207:i32)  [unwired: 4 out]
          n92 = case shown="0, Default" w207 {
            tunnel: w206 -> [w211 w221]
            tunnel: [w210 w221] -> w205
            tunnel: w204 -> [w215 _]
            tunnel: w203 -> [w214 _]
            tunnel: w202 -> [w213 _]
            frame 0, Default {
              n93 = call "Split_Ch_name.vi"("Ch name"=w213) -> ("Low level"=w217:string)  [unwired: 2 out]
              n94 = Number To Fractional String(number=w215, precision (6)=i16 3) -> (F-format string=w220:string)  [unwired: 2 out]
              n95 = Number To Fractional String(number=w214, precision (6)=i16 1) -> (F-format string=w218:string)  [unwired: 2 out]
              n96 = Build Array(w217, w220, w218) -> (w212:string[])
              n97 = Build Array (concatenate)(w211, w212) -> (w210:string[][])
            }
            frame -1 {
            }
          }
        }
        n98 = local write "Gas Remaining"(w194) -> ()
      }
      frame "Setup Continued" {
        n99 = property on="OK" class="Bool"("Key Focus"=TRUE ("Write Attribute")) -> ()  [unwired: 2 in, 2 out]
      }
      frame "Update Values" {
        n100 = for {
          tunnel: w234 -> [w241] mode=indexing
          tunnel: [w240] -> w233 mode=indexing
          tunnel: w232 -> [w239] mode=indexing
          tunnel: [w238] -> w231 mode=indexing
          tunnel: w229 -> [w237] mode=indexing
          tunnel: [w236] -> w228 mode=indexing
          n101 = Unbundle By Name(w241) -> ("Calibration type"=w244:T6, "String"=w243:string, "Ch Name"=w242:string)
          n102 = case shown="\"Text\"" w244 {
            tunnel: w243 -> [_ w265]
            tunnel: w242 -> [_ w255]
            tunnel: w241 -> [w247 w259]
            tunnel: [w247 w258] -> w240
            tunnel: w239 -> [w246 w257]
            tunnel: [w246 w256] -> w238
            tunnel: w237 -> [w245 w254]
            tunnel: [w245 w248] -> w236
            frame "Raw", Default {
            }
            frame "Text" {
              n103 = call "Get_array_values_fr_String.vi"("String Value"=w265) -> ("String array"=w252:string[])  [unwired: 1 out]
              n104 = To Unsigned Word Integer(number=w257) -> (unsigned 16bit integer=w263:u16)
              n105 = Build Array (concatenate)(w252, "Edit Strings") -> (w251:string[])
              n106 = Array Size(array=w252) -> (size(s)=w264:i32)
              n107 = case shown="\"GMU:Trace:Hi-Tec Range\"" w255 {
                tunnel: [w272 w276 w281 w286 w290 w294 w299 w304] -> w249
                tunnel: w252 -> [_ w274 w278 w284 _ _ _ _]
                tunnel: w263 -> [w272 w277 w282 w287 w291 w295 w300 w305]
                tunnel: w254 -> [_ w275 w280 w285 w289 w293 w298 w303]
                tunnel: w251 -> [_ _ _ _ _ _ w297 w302]
                frame "No match", Default {
                }
                frame "GMU:Trace:Gas" {
                  n108 = property on="Trace Gas" class="Ring (strict)"("Strings []"=w274) -> ()  [unwired: 2 in, 2 out]
                  n109 = Select(t=w277, s=w275, f="Trace Gas") -> (s? t:f=w276:u16)
                  n110 = local write "Trace Gas"(w276) -> ()
                }
                frame "GMU:Carrier 1:Gas" {
                  n111 = property on="Carrier 1 Gas" class="Ring (strict)"("Strings []"=w278) -> ()  [unwired: 2 in, 2 out]
                  n112 = Select(t=w282, s=w280, f="Carrier 1 Gas") -> (s? t:f=w281:u16)
                  n113 = local write "Carrier 1 Gas"(w281) -> ()
                }
                frame "GMU:Carrier 2:Gas" {
                  n114 = property on="Carrier 2 Gas" class="Ring (strict)"("Strings []"=w284) -> ()  [unwired: 2 in, 2 out]
                  n115 = Select(t=w287, s=w285, f="Carrier 2 Gas") -> (s? t:f=w286:u16)
                  n116 = local write "Carrier 2 Gas"(w286) -> ()
                }
                frame "GMU:Carrier 1:Hi-Tec Range" {
                  n117 = Select(t=w291, s=w289, f="Carrier 1 Hi-Tec Range") -> (s? t:f=w290:u16)
                  n118 = local write "Carrier 1 Hi-Tec Range"(w290) -> ()
                }
                frame "GMU:Trace:Hi-Tec Range" {
                  n119 = Select(t=w295, s=w293, f="Trace Hi-Tec Range") -> (s? t:f=w294:u16)
                  n120 = local write "Trace Hi-Tec Range"(w294) -> ()
                }
                frame "GMU:Source:Type" {
                  n121 = property on="Source Type" class="Ring (strict)"("Strings []"=w297) -> ()  [unwired: 2 in, 2 out]
                  n122 = Select(t=w300, s=w298, f="Source Type") -> (s? t:f=w299:u16)
                  n123 = local write "Source Type"(w299) -> ()
                }
                frame "GMU:Release:Orientation" {
                  n124 = property on="Release Orientation" class="Ring (strict)"("Strings []"=w302) -> ()  [unwired: 2 in, 2 out]
                  n125 = Select(t=w305, s=w303, f="Release Orientation") -> (s? t:f=w304:u16)
                  n126 = local write "Release Orientation"(w304) -> ()
                }
              }
              n127 = To Unsigned Word Integer(number=w264) -> (unsigned 16bit integer=w262:u16)
              n128 = Equal?(x=w262, y=w249) -> (x = y?=w248:bool)
              n129 = case shown="True" w248 {
                tunnel: w252 -> [w267 w271]
                tunnel: w255 -> [_ w270]
                tunnel: [w267 w269] -> w260
                tunnel: [w266 w268] -> w250
                tunnel: w249 -> [w266 _]
                frame False {
                }
                frame True {
                  n130 = call "Edit_String_Options_list.vi"("Channel Name"=w270, "String array"=w271) -> ("New Selection Index"=w268:i32, "String array Out"=w269:string[])
                }
              }
              n131 = call "Put_Array_into_String.vi"("String array"=w260) -> ("String Value"=w261:string)
              n132 = Bundle By Name(cluster=w259, "String"=w261) -> (w258:T2)
              n133 = To Double Precision Float(number=w250) -> (double precision float=w256:dbl)
            }
          }
        }
      }
      frame "Slow FID Calib Gas" {
        n134 = Less?(x=w308, y=10) -> (x < y?=w306:bool)
        n135 = Select(t="Initialise Hi tec selection", s=w306, f="Update Release Temperature") -> (s? t:f=w311:string)
      }
      frame "Initialise Hi tec selection" {
        n136 = local read "Carrier 1 Hi-Tec Range"() -> (w322:u16)
        n137 = local read "Trace Hi-Tec Range"() -> (w318:u16)
        n138 = case shown="2" w322 {
          tunnel: [FALSE FALSE TRUE] -> w321
          tunnel: [FALSE TRUE FALSE] -> w320
          tunnel: [TRUE FALSE FALSE] -> w319
          frame 0, Default {
          }
          frame 1 {
          }
          frame 2 {
          }
        }
        n139 = case shown="0, Default" w318 {
          tunnel: [TRUE FALSE FALSE] -> w317
          tunnel: [FALSE FALSE TRUE] -> w316
          frame 0, Default {
          }
          frame 1 {
          }
          frame 2 {
          }
        }
        n140 = local write "Carrier 1 Very Low"(w319) -> ()
        n141 = local write "Carrier 1 High"(w321) -> ()
        n142 = local write "Carrier 1 Low"(w320) -> ()
        n143 = local write "300 ml/min"(w316) -> ()
        n144 = local write "5 ml/min"(w317) -> ()
      }
      frame "Update Release Temperature" {
        n145 = while {
          tunnel: [w357] -> w348
          shift-left: _ -> [w357]
          shift-right: [w358] -> w349
          stop <- FALSE continue-if-true
          n146 = Get Date/Time In Seconds() -> (seconds since 1Jan1904=w355:timestamp)
          n147 = To Double Precision Float(number=w355) -> (double precision float=w358:dbl)
        }
        n148 = local read "Ch names"() -> (w343:string[])
        n149 = Not Equal To 0?(x="Release Temperature") -> (x != 0?=w346:bool)
        n150 = Not Equal?(x=w348, y=w349) -> (x != y?=w347:bool)
        n151 = And(x=w346, y=w347) -> (x .and. y?=w345:bool)
        n152 = case shown="True" w345 {
          tunnel: w343 -> [_ w361]
          tunnel: "Release Temperature" -> [_ w360]
          frame False {
          }
          frame True {
            n153 = Decrement(x=w360) -> (x-1=w359:u16)
            n154 = Index Array(array=w361, index=w359) -> (element=w366:string)
            n155 = Build Array(w366) -> (w365:string[])
            n156 = call "Get_Current_Scan_client.vi"("ADAM Ch Names"=w365) -> ("Numerical Values"=w363:dbl[])  [unwired: 3 out]
            n157 = Index Array(array=w363, index=0) -> (element=w362:dbl)
            n158 = local write "Current Release Temp"(w362) -> ()
          }
        }
      }
      frame "Sort out Valve Logic" {
        n159 = while {
          shift-left: _ -> [w373]
          shift-right: [w374] -> _
          shift-left: _ -> [w375]
          shift-right: [w378] -> _
          shift-left: _ -> [w376]
          shift-right: [w377] -> _
          shift-left: _ -> [w379]
          shift-right: [w381] -> _
          shift-left: _ -> [w380]
          shift-right: [w382] -> _
          stop <- FALSE continue-if-true
          n160 = stacked-sequence {
            tunnel: ["Carrier 1 High" _] -> w382
            tunnel: ["Carrier 1 Low" _] -> w381
            tunnel: w380 -> [w391 _]
            tunnel: w379 -> [w390 _]
            tunnel: [_ "300 ml/min"] -> w378
            tunnel: [_ "5 ml/min"] -> w377
            tunnel: w376 -> [_ w404]
            tunnel: w375 -> [_ w403]
            tunnel: ["Carrier 1 Very Low" _] -> w374
            tunnel: w373 -> [w385 _]
            frame #0 {
              n161 = Build Array("Carrier 1 Very Low", "Carrier 1 High", "Carrier 1 Low") -> (w389:T1[])
              n162 = Boolean To (0,1)(Boolean=w389) -> (0, 1=w388:i16[])
              n163 = Add Array Elements(numeric array=w388) -> (sum=w387:i16)
              n164 = case shown="2, Default" w387 {
                tunnel: w391 -> [_ _ w398]
                tunnel: w390 -> [_ _ w397]
                tunnel: "Carrier 1 Very Low" -> [_ _ w400]
                tunnel: w385 -> [_ _ w399]
                tunnel: "Carrier 1 Low" -> [_ _ w396]
                tunnel: "Carrier 1 High" -> [_ _ w395]
                frame 0 {
                }
                frame 1 {
                }
                frame 2, Default {
                  n165 = Exclusive Or(1:w399, 2:w400) -> (0:w394:T1)
                  n166 = Exclusive Or(1:w397, 2:w396) -> (0:w392:T1)
                  n167 = Exclusive Or(1:w398, 2:w395) -> (0:w393:T1)
                  n168 = local write "Carrier 1 Very Low"(w394) -> ()
                  n169 = local write "Carrier 1 High"(w393) -> ()
                  n170 = local write "Carrier 1 Low"(w392) -> ()
                }
              }
            }
            frame #1 {
              n171 = Build Array("5 ml/min", "300 ml/min") -> (w407:T1[])
              n172 = Boolean To (0,1)(Boolean=w407) -> (0, 1=w406:i16[])
              n173 = Add Array Elements(numeric array=w406) -> (sum=w405:i16)
              n174 = case shown="2, Default" w405 {
                tunnel: w404 -> [_ _ w413]
                tunnel: w403 -> [_ _ w412]
                tunnel: "300 ml/min" -> [_ _ w411]
                tunnel: "5 ml/min" -> [_ _ w410]
                frame 0 {
                }
                frame 1 {
                }
                frame 2, Default {
                  n175 = Exclusive Or(1:w412, 2:w411) -> (0:w408:T1)
                  n176 = Exclusive Or(1:w413, 2:w410) -> (0:w409:T1)
                  n177 = local write "300 ml/min"(w408) -> ()
                  n178 = local write "5 ml/min"(w409) -> ()
                }
              }
            }
          }
        }
      }
      frame "Hi Tec Ranges" {
        n179 = local read "Carrier 1 Very Low"() -> (w415:T1)
        n180 = local read "5 ml/min"() -> (w416:T1)
        n181 = case shown="False" w415 {
          tunnel: [w425 u16 0 ("Carrier 1 Hi-Tec Range")] -> w414
          frame False {
            n182 = local read "Carrier 1 Low"() -> (w426:T1)
            n183 = Select(t=u16 1 ("Carrier 1 Hi-Tec Range"), s=w426, f=u16 2 ("Carrier 1 Hi-Tec Range")) -> (s? t:f=w425:u16)
          }
          frame True {
          }
        }
        n184 = case shown="False" w416 {
          tunnel: [u16 2 ("Carrier 1 Hi-Tec Range") u16 0 ("Carrier 1 Hi-Tec Range")] -> w417
          frame False {
          }
          frame True {
          }
        }
        n185 = local write "Carrier 1 Hi-Tec Range"(w414) -> ()
        n186 = local write "Trace Hi-Tec Range"(w417) -> ()
      }
      frame "Continue looping?" {
        n187 = local read "Select Plug Ins"() -> (w431:bool)
        n188 = Compound Arithmetic op=OR("stop", "OK", w431) -> (w430:bool)
        n189 = Current VI's Path() -> (path=w438:path)
        n190 = call "Close_Panel_and_Abort.vi"("Vi path"=w438, "stop"="stop") -> ()  [unwired: 1 out]
        n191 = Select(t="Insert Values", s=w430, f="Update Values") -> (s? t:f=w435:string)
      }
      frame "Insert Values" {
        n192 = local read "Ch names"() -> (w442:string[])
        n193 = for {
          tunnel: w444 -> [w452] mode=indexing
          tunnel: w445 -> [w454] mode=indexing
          tunnel: [w453] -> w446 mode=indexing
          tunnel: [w451] -> w443 mode=indexing
          tunnel: w442 -> [w450]
          n194 = Unbundle By Name(w452) -> ("Ch Name"=w455:string)
          n195 = case shown="\"GMU:Source:Release Temp\"" w455 {
            tunnel: w454 -> [_ _ _ w476]
            tunnel: [w456 w458 w460 w476] -> w453
            tunnel: w452 -> [w457 w459 w464 w475]
            tunnel: [w457 w459 w463 w475] -> w451
            tunnel: w450 -> [_ _ w462 _]
            frame "GMU:Calibration:Gas 1" {
              n196 = local read "Calib 1"() -> (w456:dbl)
            }
            frame "GMU:Calibration:Gas 2" {
              n197 = local read "Calib 2"() -> (w458:dbl)
            }
            frame "GMU:Source:Release Temp" {
              n198 = local read "Release Temperature"() -> (w461:u16)
              n199 = Equal To 0?(x=w461) -> (x = 0?=w467:bool)
              n200 = case shown="True" w467 {
                tunnel: w461 -> [w469 _]
                tunnel: w462 -> [w472 _]
                tunnel: [w471 ""] -> w465
                tunnel: [w470 w473] -> w466
                frame False {
                  w470 = T3 "Read Ch"  # Module Type
                  n201 = Decrement(x=w469) -> (x-1=w468:u16)
                  n202 = Index Array(array=w472, index=w468) -> (element=w471:string)
                }
                frame True {
                  w473 = T3 "Hold Value"  # Module Type
                }
              }
              n203 = local read "Current Release Temp"() -> (w460:dbl)
              n204 = Bundle By Name(cluster=w464, "String"=w465, "Type"=w466) -> (w463:T2)
            }
            frame "No Match", Default {
            }
          }
        }
      }
      frame "Insert Gas Remaining Info" {
        n205 = local read "Gas Remaining"() -> (w482:string[][])
        n206 = Index Array(array=w482, index (col)=0 ("disabled index (col)")) -> (element=w478:string[])  [unwired: 1 in]
        n207 = for {
          tunnel: w479 -> [w492]
          tunnel: w478 -> [w491] mode=indexing
          tunnel: [w490] -> w477 mode=indexing
          n208 = Concatenate Strings(w492, w491) -> (w490:string)
        }
        n209 = Index Array(array=w482, index (col)=1 ("disabled index (col)")) -> (element=w481:string[])  [unwired: 1 in]
        n210 = for {
          tunnel: w480 -> [w505] mode=indexing
          tunnel: w485 -> [w493] mode=indexing
          tunnel: [w501] -> w486 mode=indexing
          tunnel: w477 -> [w504]
          tunnel: w481 -> [w502]
          n211 = Unbundle By Name(w505) -> ("Ch Name"=w503:string)
          n212 = Search 1D Array(1D array=w504, element=w503) -> (index of element=w499:i32)  [unwired: 1 out]
          n213 = Number To Fractional String(number=w493, precision (6)=i16 3) -> (F-format string=w497:string)  [unwired: 2 out]
          n214 = Index Array(array=w502, index=w499) -> (element=w498:string)
          n215 = Greater Or Equal To 0?(x=w499) -> (x >= 0?=w496:bool)
          n216 = Not Equal?(x=w497, y=w498) -> (x != y?=w495:bool)
          n217 = And(x=w495, y=w496) -> (x .and. y?=w494:bool)
          n218 = case shown="False" w494 {
            tunnel: [w506 w508] -> w501
            tunnel: w498 -> [_ w507]
            tunnel: w493 -> [w506 _]
            frame False {
            }
            frame True {
              n219 = Fract/Exp String To Number(string=w507) -> (number=w508:dbl)  [unwired: 4 out]
            }
          }
        }
      }
      frame "Insert Source info values" {
        n220 = for {
          tunnel: w512 -> [w529] mode=indexing
          tunnel: [w528] -> w520 mode=indexing
          n221 = Unbundle By Name(w529) -> ("Ch Name"=w528:string)
        }
        n222 = Index Array(array="Source Info", index (col)=0 ("disabled index (col)")) -> (element=w516:string[])  [unwired: 1 in]
        n223 = Index Array(array="Source Info", index (col)=1 ("disabled index (col)")) -> (element=w513:string[])  [unwired: 1 in]
        n224 = for {
          tunnel: w520 -> [w527]
          tunnel: w516 -> [w526] mode=indexing
          shift-right: [w523] -> w514
          shift-left: w515 -> [w524]
          tunnel: w513 -> [w522] mode=indexing
          n225 = Fract/Exp String To Number(string=w522) -> (number=w521:dbl)  [unwired: 4 out]
          n226 = Search 1D Array(1D array=w527, element=w526) -> (index of element=w525:i32)  [unwired: 1 out]
          n227 = Replace Array Subset(array=w524, new element=w521, index=w525) -> (w523:dbl[])
        }
      }
      frame "Update Server" {
        w535 = T10 {"Channel Name"="", "New Value"=0.0} ("Update Scan Value Cluster")
        n228 = Index Array(array=w540, index=0 ("Index")) -> (element=w551:T2)
        n229 = local read "Ch Description Array"() -> (w537:T2[])
        n230 = local read "Numerical Values"() -> (w536:dbl[])
        n231 = Initialize Array(w551, 0 ("Dimension Size")) -> (w549:T2[])
        n232 = Initialize Array(w535, 0 ("Dimension Size")) -> (w544:T10[])
        n233 = for {
          shift-right: [w564] -> w546
          shift-left: w549 -> [w565]
          tunnel: w540 -> [w555] mode=indexing
          shift-right: [w563] -> w541
          shift-left: w544 -> [w562]
          tunnel: w539 -> [w557] mode=indexing
          tunnel: w537 -> [w556] mode=indexing
          tunnel: w536 -> [w560] mode=indexing
          tunnel: w535 -> [w558]
          n234 = Equal?(x=w555, y=w556) -> (x = y?=w561:bool)
          n235 = Equal?(x=w557, y=w560) -> (x = y?=w559:bool)
          n236 = case shown="False" w559 {
            tunnel: w562 -> [w572 w573]
            tunnel: [w571 w573] -> w563
            tunnel: w558 -> [w570 _]
            tunnel: w557 -> [w569 _]
            tunnel: w555 -> [w568 _]
            frame False {
              n237 = Unbundle By Name(w568) -> ("Ch Name"=w567:string)
              n238 = Bundle By Name(cluster=w570, "Channel Name"=w567, "New Value"=w569) -> (w566:T10)
              n239 = Build Array (concatenate)(w572, w566) -> (w571:T10[])
            }
            frame True {
            }
          }
          n240 = case shown="True" w561 {
            tunnel: w565 -> [w576 w577]
            tunnel: w555 -> [w575 _]
            tunnel: [w574 w577] -> w564
            frame False {
              n241 = Build Array (concatenate)(w576, w575) -> (w574:T2[])
            }
            frame True {
            }
          }
        }
        n242 = Array Size(array=w546) -> (size(s)=w548:i32)
        n243 = Array Size(array=w541) -> (size(s)=w542:i32)
        n244 = Greater Than 0?(x=w548) -> (x > 0?=w547:bool)
        n245 = Greater Than 0?(x=w542) -> (x > 0?=w543:bool)
        n246 = case shown="True" w547 {
          tunnel: w546 -> [_ w554]
          frame False {
          }
          frame True {
            n247 = call "Update_Ch_Discription_client.vi"("Channels to update In"=w554) -> ()  [unwired: 1 out]
          }
        }
        n248 = case shown="True" w543 {
          tunnel: w541 -> [_ w553]
          frame False {
          }
          frame True {
            n249 = call "Update_Current_Value_client.vi"("Update array in"=w553) -> ()  [unwired: 1 in]
          }
        }
        n250 = Select(t="Select Server Channels", s="Select Plug Ins", f="Close Panel") -> (s? t:f=w531:string)
      }
      frame "Select Server Channels" {
        w581 = string[] []
        w590 = T11."Zero or more"  # Selector mode
        n251 = local read "Source Info"() -> (w588:string[][])
        n252 = global read "Preference_global.vi" "Rig Setup"() -> (w601:string)
        n253 = Concatenate Strings(w601, ":" ("string")) -> (w598:string)
        n254 = String Length(string=w598) -> (length=w599:i32)
        n255 = call "Get_ADAM_Ch_names_client.vi"("Channel names set"=Channel_names."All Channels") -> ("Ch names"=w591:string[])
        n256 = Index Array(array=w588, index (col)=0) -> (element=w583:string[])  [unwired: 1 in]
        n257 = for {
          tunnel: w599 -> [w634]
          tunnel: w591 -> [w624] mode=indexing
          tunnel: w598 -> [w626]
          shift-right: [w628] -> w589
          shift-left: string[] [] -> [w629]
          n258 = Search/Split String(string=w624, offset (0)=w634) -> (substring before match=w633:string, match + rest of string=w632:string)  [unwired: 2 out]
          n259 = Equal?(x=w626, y=w633) -> (x = y?=w622:bool)
          n260 = Match Pattern(string=w632, regular expression="[Ss]ource") -> (offset past match=w630:i32)  [unwired: 4 out]
          n261 = Concatenate Strings(w626, "Source:Status") -> (w625:string)
          n262 = Greater Or Equal To 0?(x=w630) -> (x >= 0?=w623:bool)
          n263 = Equal?(x=w625, y=w624) -> (x = y?=w621:bool)
          n264 = Compound Arithmetic op=AND(invert w621, w622, w623) -> (w620:bool)
          n265 = case shown="True" w620 {
            tunnel: w629 -> [w635 w638]
            tunnel: w624 -> [_ w636]
            tunnel: [w635 w637] -> w628
            frame False {
            }
            frame True {
              n266 = Build Array (concatenate)(w638, w636) -> (w637:string[])
            }
          }
        }
        n267 = call "Select_Strings.vi"("Available Ch names"=w589, "Message"="Please select the appropriate source information channels", "Selector mode"=w590, "Desired Ch names (in)"=w583) -> ("Selected Channel Names"=w582:string[])  [unwired: 1 in, 3 out]
        n268 = for {
          tunnel: w583 -> [w605] mode=indexing
          tunnel: w582 -> [w606]
          shift-right: [w602] -> w580
          shift-left: w581 -> [w603]
          n269 = Search 1D Array(1D array=w606, element=w605) -> (index of element=w604:i32)  [unwired: 1 out]
          n270 = case shown="-1" w604 {
            tunnel: w605 -> [_ w610]
            tunnel: w603 -> [w607 w609]
            tunnel: [w607 w608] -> w602
            frame 0, Default {
            }
            frame -1 {
              n271 = Build Array (concatenate)(w609, w610) -> (w608:string[])
            }
          }
        }
        n272 = call "Adam_Ch_on_off.vi"("Ch State"=Channel_State."Always Off", "ADAM Ch Names"=w580) -> ()  [unwired: 1 out]
        n273 = for {
          tunnel: w582 -> [w614] mode=indexing
          tunnel: w583 -> [w615]
          shift-right: [w611] -> w584
          shift-left: w581 -> [w612]
          n274 = Search 1D Array(1D array=w615, element=w614) -> (index of element=w613:i32)  [unwired: 1 out]
          n275 = case shown="-1" w613 {
            tunnel: w614 -> [_ w619]
            tunnel: w612 -> [w616 w618]
            tunnel: [w616 w617] -> w611
            frame 0, Default {
            }
            frame -1 {
              n276 = Build Array (concatenate)(w618, w619) -> (w617:string[])
            }
          }
        }
        n277 = call "Adam_Ch_on_off.vi"("Ch State"=Channel_State."On", "ADAM Ch Names"=w584) -> ()  [unwired: 1 out]
      }
      frame "Close Panel" {
        n278 = local read "dup reference"() -> (w640:refnum<vi>)
        n279 = property class="VI"(reference=w640, "Front Panel Window:Open"=FALSE) -> (reference out=w642:refnum<vi>, error out=w641:errorcluster)  [unwired: 1 in]
        n280 = Close Reference(reference=w642, error in (no error)=w641) -> ()  [unwired: 1 out]
      }
    }
  }
